vi "snapRectangle.vi"(0 "reference":refnum<class "Grid.lvclass">, 1 "bounds":T1 {"height" format="%.2f"; "width" format="%.2f"; "y" format="%.2f"; "x" format="%.2f"}, 5 "error in (no error)":errorcluster) -> (14 "reference out":refnum<class "Grid.lvclass">, 15 "boundsOut":T1 {"height" format="%.2f"; "width" format="%.2f"; "y" format="%.2f"; "x" format="%.2f"}, 19 "error out":errorcluster)   [LabVIEW 2012, in "Grid.lvclass"]
doc: "public void snap(Rectangle2D r)"
uses:
  <resource>/Framework/Providers/Open_GDS/UML/Grid_class/Grid.lvclass
  <resource>/Framework/Providers/Open_GDS/UML/General/Rectangle/Rectangle Rectangle2D.ctl
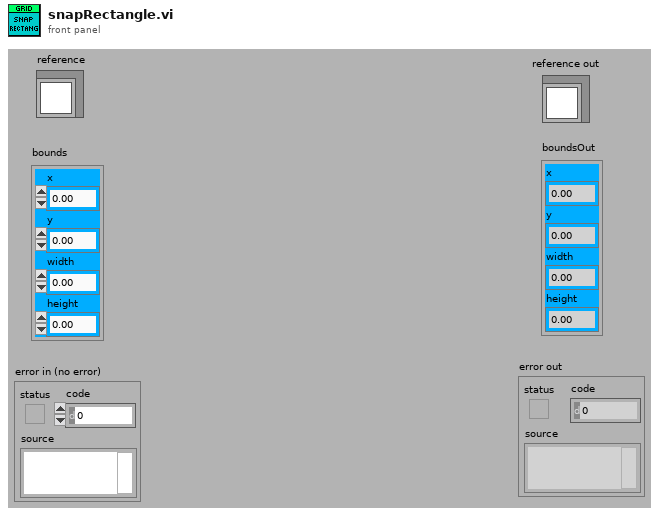
[diagram p1: front panel]
types:
  T1 = typedef "Rectangle Rectangle2D.ctl" = cluster{"x":dbl, "y":dbl, "width":dbl, "height":dbl}
  T2 = typedef "Grid.lvclass/ObjectAttributes.ctl" = cluster{"gridX":dbl, "gridY":dbl, "gridColor":u32}
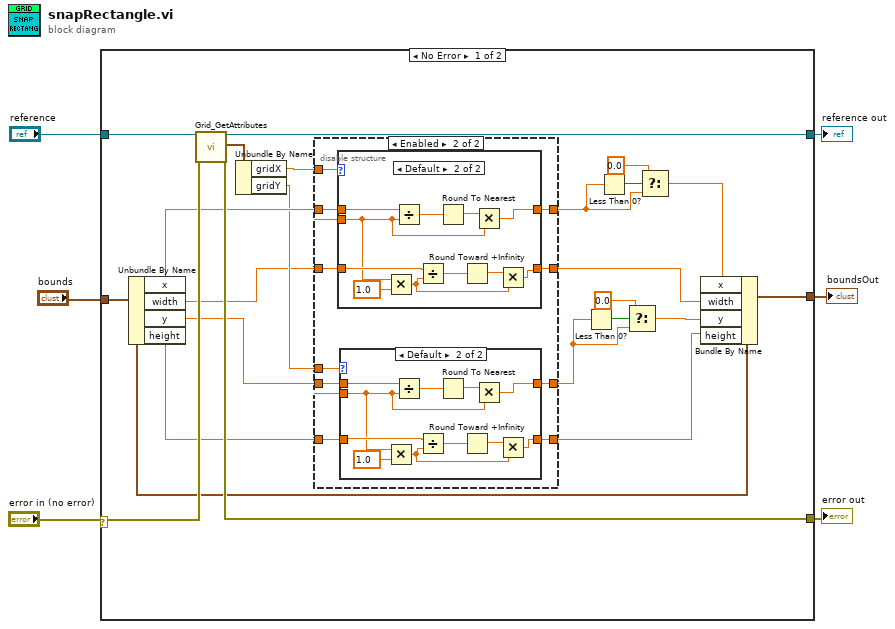
[diagram p0: block diagram]
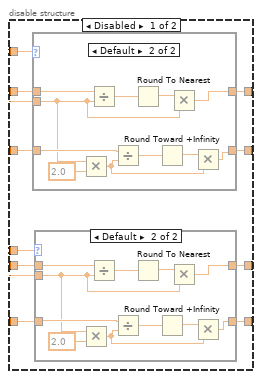
[diagram p2: hidden frame]
diagram:
  n1 = case shown="No Error" "error in (no error)" {
    selector: "error in (no error)" -> [w26 w102]
    tunnel: "reference" -> [w29 w103]
    tunnel: [w28 w102] -> w5
    tunnel: [w27 w103] -> w4
    tunnel: "bounds" -> [w25 _]
    tunnel: [w15 _] -> w1
    frame No Error {
      n2 = Unbundle By Name(w25) -> ("x"=w24:dbl, "width"=w19:dbl, "y"=w21:dbl, "height"=w18:dbl)
      n3 = call <resource>:"Grid_GetAttributes.vi"("reference in"=w29, "error in (no error)"=w26) -> ("reference out"=w27:refnum<class "Grid.lvclass">, "Attributes"=w20:T2, "error out"=w28:errorcluster)  [unwired: 15 out]
      n4 = Unbundle By Name(w20) -> ("gridX"=w23:dbl, "gridY"=w22:dbl)
      n5 = disable-structure shown="Enabled" {
        disable-tunnel: w24 -> [w39 w75]
        disable-tunnel: w23 -> [w38 w74]
        disable-tunnel: w22 -> [w37 w73]
        disable-tunnel: w21 -> [w36 w72]
        disable-tunnel: w19 -> [w35 w71]
        disable-tunnel: w18 -> [w34 w70]
        disable-tunnel: [w33 w69] -> w17
        disable-tunnel: [w32 w68] -> w16
        disable-tunnel: [w31 w67] -> w11
        disable-tunnel: [w30 w66] -> w7
        frame Disabled {
          n6 = case shown="Default" w38 {
            tunnel: w39 -> [w54 w65]
            tunnel: w38 -> [_ w57]
            tunnel: [w54 w62] -> w31
            tunnel: w35 -> [w53 w58]
            tunnel: [w53 w55] -> w32
            frame 0 {
            }
            frame Default {
              n7 = Multiply(x=w57, y=2.0) -> (x*y=w61:dbl)
              n8 = Divide(x=w65, y=w57) -> (x/y=w64:dbl)
              n9 = Divide(x=w58, y=w61) -> (x/y=w59:dbl)
              n10 = Round To Nearest(number=w64) -> (nearest integer value=w63:dbl)
              n11 = Round Toward +Infinity(x=w59) -> (ceil(x): smallest int >= x=w60:dbl)
              n12 = Multiply(x=w63, y=w57) -> (x*y=w62:dbl)
              n13 = Multiply(x=w60, y=w61) -> (x*y=w55:dbl)
            }
          }
          n14 = case shown="Default" w37 {
            tunnel: w36 -> [w41 w52]
            tunnel: w37 -> [_ w42]
            tunnel: [w41 w49] -> w30
            tunnel: w34 -> [w40 w43]
            tunnel: [w40 w44] -> w33
            frame 0 {
            }
            frame Default {
              n15 = Multiply(x=w42, y=2.0) -> (x*y=w45:dbl)
              n16 = Divide(x=w52, y=w42) -> (x/y=w51:dbl)
              n17 = Divide(x=w43, y=w45) -> (x/y=w47:dbl)
              n18 = Round To Nearest(number=w51) -> (nearest integer value=w50:dbl)
              n19 = Round Toward +Infinity(x=w47) -> (ceil(x): smallest int >= x=w46:dbl)
              n20 = Multiply(x=w50, y=w42) -> (x*y=w49:dbl)
              n21 = Multiply(x=w46, y=w45) -> (x*y=w44:dbl)
            }
          }
        }
        frame Enabled {
          n22 = case shown="Default" w74 {
            tunnel: w75 -> [w90 w101]
            tunnel: w74 -> [_ w93]
            tunnel: [w90 w98] -> w67
            tunnel: w71 -> [w89 w94]
            tunnel: [w89 w91] -> w68
            frame 0 {
            }
            frame Default {
              n23 = Multiply(x=w93, y=1.0) -> (x*y=w97:dbl)
              n24 = Divide(x=w101, y=w93) -> (x/y=w100:dbl)
              n25 = Divide(x=w94, y=w97) -> (x/y=w95:dbl)
              n26 = Round To Nearest(number=w100) -> (nearest integer value=w99:dbl)
              n27 = Round Toward +Infinity(x=w95) -> (ceil(x): smallest int >= x=w96:dbl)
              n28 = Multiply(x=w99, y=w93) -> (x*y=w98:dbl)
              n29 = Multiply(x=w96, y=w97) -> (x*y=w91:dbl)
            }
          }
          n30 = case shown="Default" w73 {
            tunnel: w72 -> [w77 w88]
            tunnel: w73 -> [_ w78]
            tunnel: [w77 w85] -> w66
            tunnel: w70 -> [w76 w79]
            tunnel: [w76 w80] -> w69
            frame 0 {
            }
            frame Default {
              n31 = Multiply(x=w78, y=1.0) -> (x*y=w81:dbl)
              n32 = Divide(x=w88, y=w78) -> (x/y=w87:dbl)
              n33 = Divide(x=w79, y=w81) -> (x/y=w83:dbl)
              n34 = Round To Nearest(number=w87) -> (nearest integer value=w86:dbl)
              n35 = Round Toward +Infinity(x=w83) -> (ceil(x): smallest int >= x=w82:dbl)
              n36 = Multiply(x=w86, y=w78) -> (x*y=w85:dbl)
              n37 = Multiply(x=w82, y=w81) -> (x*y=w80:dbl)
            }
          }
        }
      }
      n38 = Less Than 0?(x=w7) -> (x < 0?=w9:bool)
      n39 = Less Than 0?(x=w11) -> (x < 0?=w14:bool)
      n40 = Select(t=0.0, s=w9, f=w7) -> (s? t:f=w8:dbl)
      n41 = Select(t=0.0, s=w14, f=w11) -> (s? t:f=w12:dbl)
      n42 = Bundle By Name(cluster=w25, "x"=w12, "width"=w16, "y"=w8, "height"=w17) -> (w15:T1)
    }
    frame Error {
    }
  }
  "reference out" <- w4
  "error out" <- w5
  "boundsOut" <- w1
